vi "manifest.vi"() -> ()   [LabVIEW 2014]
panel:
  in  "logService.vi":T1={"标题"="日志服务", "相对路径"="service\\logService.vi", "类型"=enum."服务", "专属队列名称"="23jw1drSUhlT873VYsPws58raxR0Wi"}
  in  "main.vi":T1={"标题"="UAES", "相对路径"="main.vi", "类型"=enum."活动", "专属队列名称"="uwIU53LgK50HLoFSAGWrIyzrfdcyc8"}
  in  "1_日志文件名称":string="日志文件PC"
  in  "1_日志文件储存位置":string="log"
  in  "0_程序信息":T2={"版本号"="1.0.0", "版本"="1", "版本名称"="Phoenix", "单位网络地址"="http://www.doe.zju.edu.cn/vehicle", "程序名称"="车载测试程序", "开发方单位名称"="浙江大学动力机械及车辆工程研究所"}
  in  "0_消息模板":cluster{"消息":string, "数据":variant}
  in  "activity模板.vi":T1={"标题"="未命名", "相对路径"="R\\activity模板.vi", "类型"=enum."活动", "专属队列名称"="yQPC7c1ByUa59utYbVeowZ9iPz3wrH"}
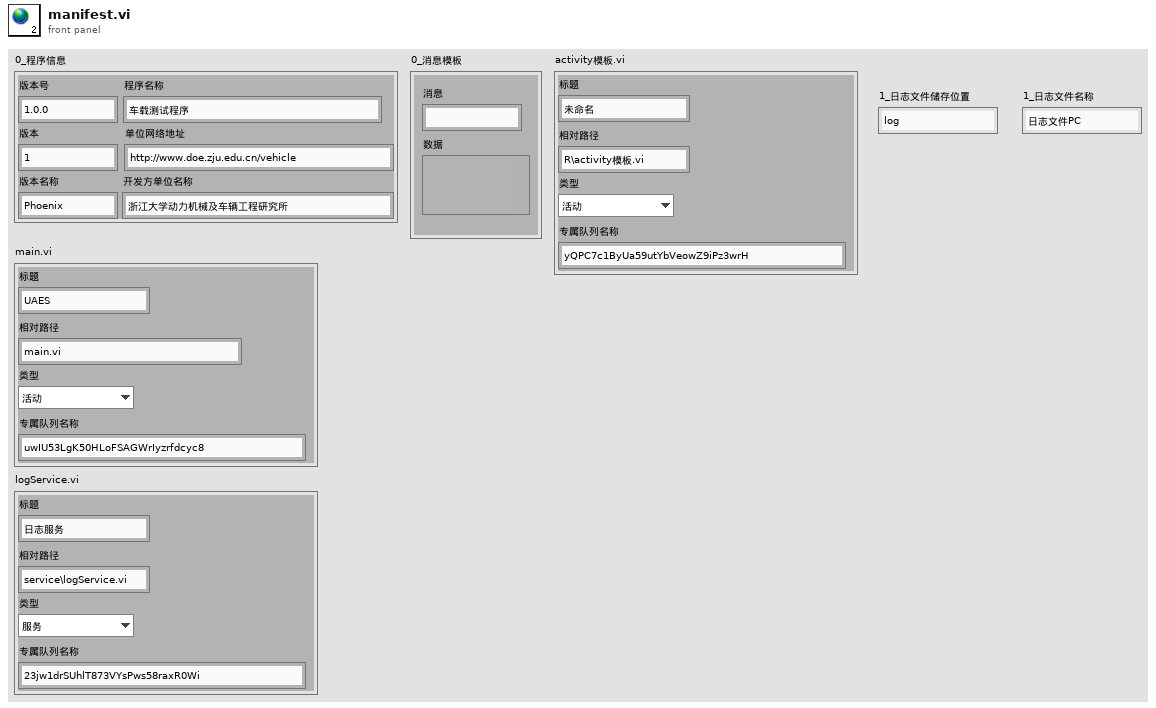
[diagram p1: front panel]
types:
  T1 = cluster{"标题":string, "相对路径":string, "类型":enum16{"服务", "活动"}, "专属队列名称":string}
  T2 = cluster{"版本号":string, "版本":string, "版本名称":string, "单位网络地址":string, "程序名称":string, "开发方单位名称":string}
diagram:
